vi "Write MXN.vi"(8 "error in (no error)":errorcluster, 10 "MXN":bool, 11 "Nestle  Actor in":refnum<class "Nestle  Actor.lvclass">) -> (0 "error out":errorcluster, 3 "Nestle  Actor out":refnum<class "Nestle  Actor.lvclass">)   [LabVIEW 2020, in "Nestle  Actor.lvlib" / "Nestle  Actor.lvclass"]
uses:
  Nestle  Actor.lvclass
  Nestle  Actor.lvclass/Nestle  Actor.ctl
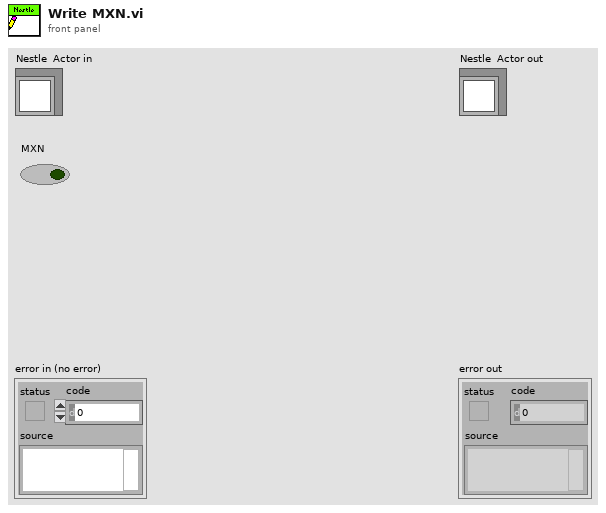
[diagram p1: front panel]
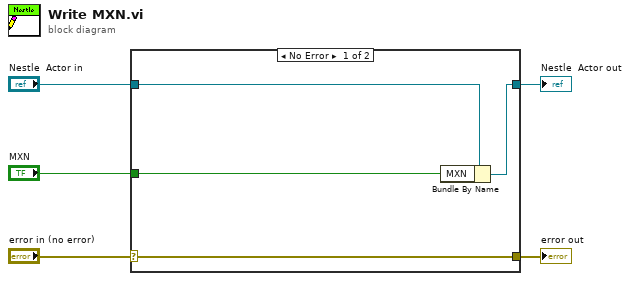
[diagram p0: block diagram]
diagram:
  n1 = case shown="No Error" "error in (no error)" {
    selector: "error in (no error)" -> [w9 w10]
    tunnel: [w9 w10] -> w4
    tunnel: [w7 w11] -> w2
    tunnel: "Nestle  Actor in" -> [w8 w11]
    tunnel: "MXN" -> [w6 _]
    frame No Error {
      n2 = Bundle By Name(cluster=w8, "MXN"=w6) -> (w7:refnum<class "Nestle  Actor.lvclass">)
    }
    frame Error {
    }
  }
  "error out" <- w4
  "Nestle  Actor out" <- w2
